vi "GV_UpdateLive.vi"(8 "error in (no error)":errorcluster, 9 "GviewerUpdate":T1, 11 "Gviewer in":refnum<class "Gviewer.lvclass">) -> (0 "error out":errorcluster, 1 "RollTime?":bool, 3 "Gviewer out":refnum<class "Gviewer.lvclass">)   [LabVIEW 2020, in "Sgraph_lib_V1.lvlib" / "Gviewer.lvclass"]
doc: "Andre Koelewijn, 24 April 2021\n\nThis VI will check if the life update needs to scroll the time scale together with the time (standard showing scroll view) of only update the graph (scope view)"
uses:
  Gviewer.lvclass
  FAMM/controls/FAMM_reply_datagram.ctl
  controls/Typedef_Live.ctl
  FAMM/controls/FAMM_reply_WAQdata.ctl
  FAMM/controls/FAMM_reply_EAQdata.ctl
  FAMM/controls/FAMM_reply_PAQdata.ctl
  Gviewer.lvclass/Gviewer.ctl
  FAMM/FAMM.lvclass
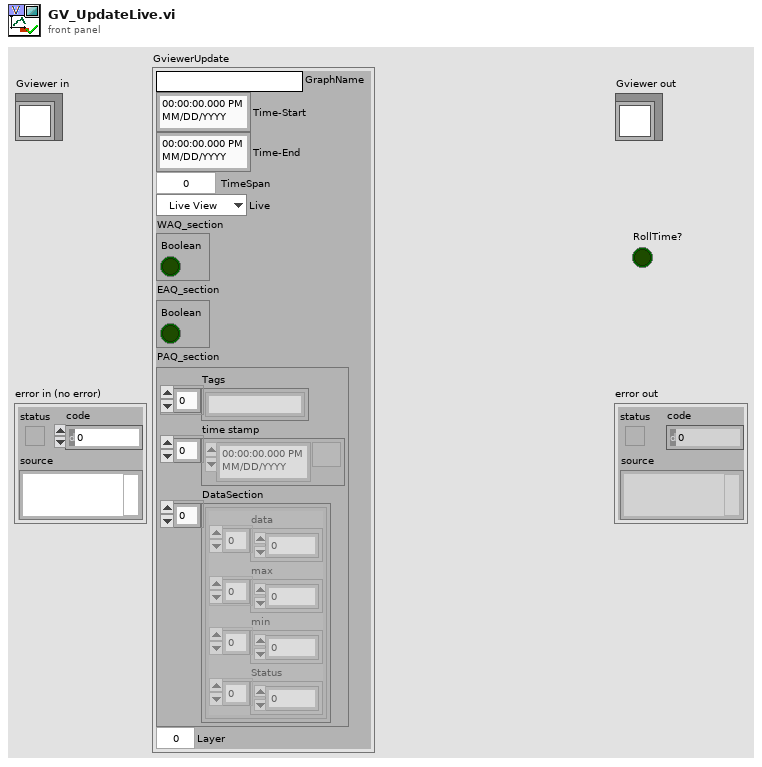
[diagram p1: front panel]
types:
  T1 = typedef "Sgraph_lib_V1.lvlib/FAMM.lvclass/FAMM_reply_datagram.ctl" = cluster{"GraphName":string, "Time-Start":timestamp, "Time-End":timestamp, "TimeSpan":dbl, "Live":T2, "WAQ_section":T3, "EAQ_section":T4, "PAQ_section":T5, "Layer":i32}
  T2 = typedef "Sgraph_lib_V1.lvlib/Gviewer.lvclass/Typedef_Live.ctl" = enum16{"Live View", "Freeze"}
  T3 = typedef "Sgraph_lib_V1.lvlib/FAMM.lvclass/FAMM_reply_WAQdata.ctl" = cluster{"Boolean":bool}
  T4 = typedef "Sgraph_lib_V1.lvlib/FAMM.lvclass/FAMM_reply_EAQdata.ctl" = cluster{"Boolean":bool}
  T5 = typedef "Sgraph_lib_V1.lvlib/FAMM.lvclass/FAMM_reply_PAQdata.ctl" = cluster{"Tags":string[], "time stamp":timestamp[], "DataSection":cluster{"data":dbl[], "max":dbl[], "min":dbl[], "Status":u32[]}[]}
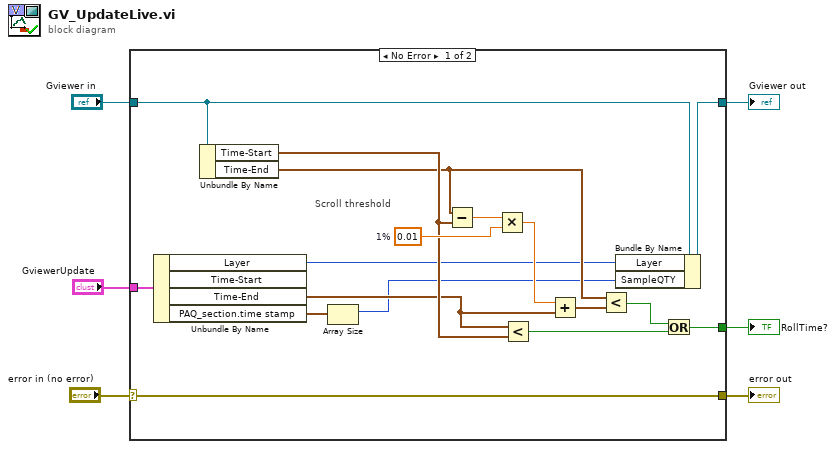
[diagram p0: block diagram]
diagram:
  n1 = case shown="No Error" "error in (no error)" {
    selector: "error in (no error)" -> [w23 w25]
    tunnel: [w23 w25] -> w5
    tunnel: [w10 w24] -> w3
    tunnel: "Gviewer in" -> [w9 w24]
    tunnel: "GviewerUpdate" -> [w12 _]
    tunnel: [w16 _] -> w1
    frame No Error {
      w21 = 0.01  # 1%
      # "Scroll threshold"
      n2 = Unbundle By Name(w12) -> ("Layer"=w11:i32, "Time-End"=w15:timestamp, "PAQ_section.time stamp"=w8:timestamp[])  [unwired: 1 out]
      n3 = Unbundle By Name(w9) -> ("Time-Start"=w17:timestamp, "Time-End"=w13:timestamp)
      n4 = Array Size(array=w8) -> (size(s)=w7:i32)
      n5 = Subtract(x=w13, y=w17) -> (x-y=w22:dbl)
      n6 = Multiply(x=w22, y=w21) -> (x*y=w20:dbl)
      n7 = Less?(x=w15, y=w17) -> (x < y?=w18:bool)
      n8 = Add(x=w20, y=w15) -> (x+y=w14:timestamp)
      n9 = Less?(x=w13, y=w14) -> (x < y?=w19:bool)
      n10 = Bundle By Name(cluster=w9, "Layer"=w11, "SampleQTY"=w7) -> (w10:refnum<class "Gviewer.lvclass">)
      n11 = Or(x=w19, y=w18) -> (x .or. y?=w16:bool)
    }
    frame Error {
    }
  }
  "error out" <- w5
  "Gviewer out" <- w3
  "RollTime?" <- w1
